vi "Test Write Pin.vi"(8 "error in (no error)":errorcluster, 11 "TestCase in":refnum<class "Test Write Port.lvclass">) -> (0 "error out":errorcluster, 3 "TestCase out":refnum<class "Test Write Port.lvclass">)   [LabVIEW 2020, in "Test Write Port.lvclass"]
uses:
  Test Write Port.lvclass
  <vilib>/addons/_JKI Toolkits/VI Tester/TestCase.llb/TestCase.lvclass
  C:/Program Files (x86)/National Instruments/LabVIEW 2020/vi.lib/addons/_JKI Toolkits/VI Tester/TestCase.llb/TestCase.lvclass
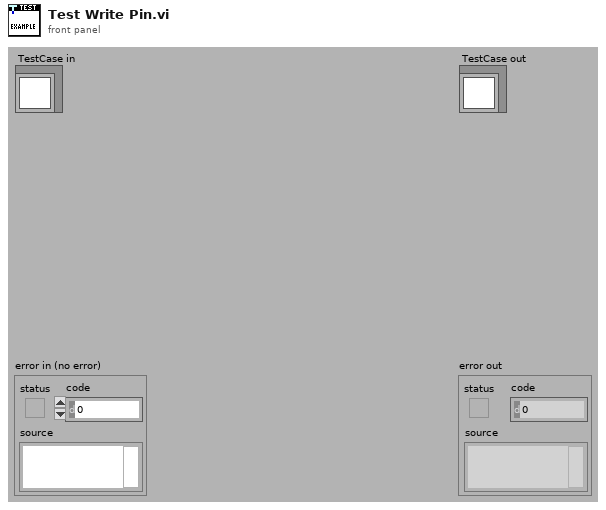
[diagram p1: front panel]
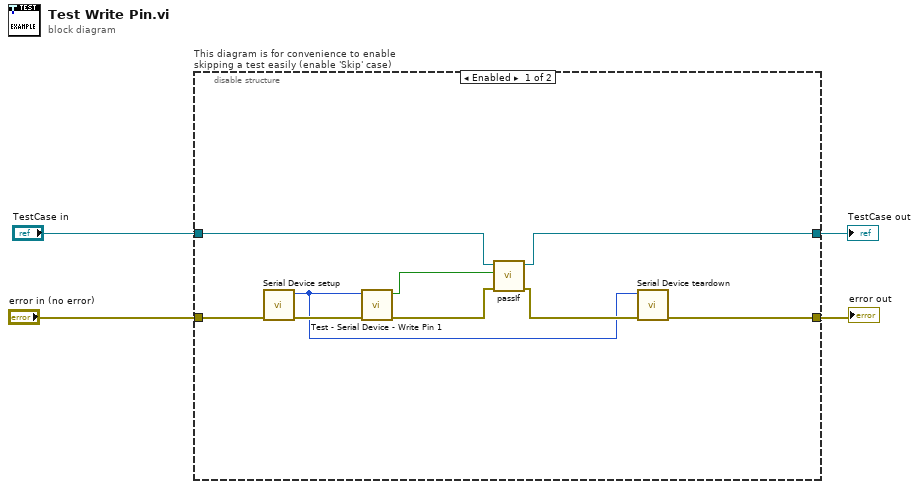
[diagram p0: block diagram]
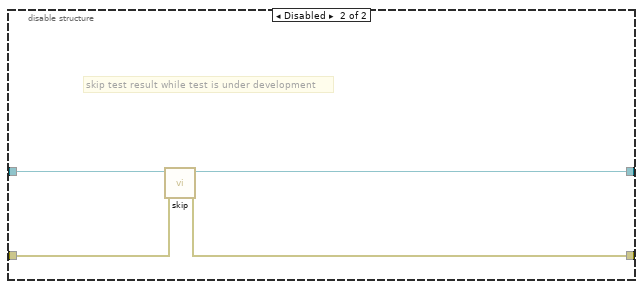
[diagram p2: hidden frame]
diagram:
  n1 = disable-structure "This diagram is for convenience to enable skipping a test easily (enable 'Skip' case)" shown="Enabled" {
    disable-tunnel: "TestCase in" -> [w13 w17]
    disable-tunnel: [w12 w15] -> w1
    disable-tunnel: [w9 w16] -> w3
    disable-tunnel: "error in (no error)" -> [w11 w14]
    frame Enabled {
      n2 = call "Serial Device setup.vi"("error in (no error)"=w11) -> ("error out"=w8:errorcluster, "Module ID"=w5:i32)  [unwired: 9 in]
      n3 = call "Test - Serial Device - Write Pin 1.vi"("error in (no error)"=w8, "Module ID"=w5) -> ("error out"=w7:errorcluster, "Pass"=w6:bool)  [unwired: 8 in]
      n4 = call-dynamic "passIf.vi"("error in (no error)"=w7, "pass"=w6, "TestCase in"=w13) -> ("error out"=w10:errorcluster, "TestCase out"=w12:refnum<class "Test Write Port.lvclass">)  [unwired: 7 in]
      n5 = call "Serial Device teardown.vi"("error in (no error)"=w10, "Module ID"=w5) -> ("error out"=w9:errorcluster)  [unwired: 9 in]
    }
    frame Disabled {
      # "skip test result while test is under development"
      n6 = call <vilib>:"skip.vi"("error in (no error)"=w14, "TestCase in"=w17) -> ("error out"=w16:errorcluster, "TestCase out"=w15:refnum<class "Test Write Port.lvclass">)  [unwired: 8 in]
    }
  }
  "error out" <- w3
  "TestCase out" <- w1
